vi "Subvi sample and hold bool.vi"(6 "Reset":bool, 8 "Refresh":bool, 9 "Input":bool) -> (1 "Output":bool)   [LabVIEW 2017]
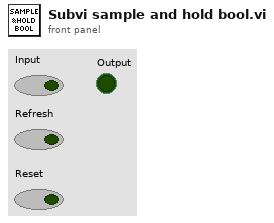
[diagram p1: front panel]
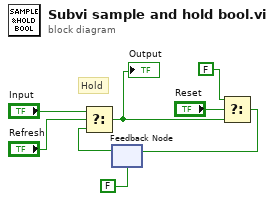
[diagram p0: block diagram]
diagram:
  # "Hold"
  n1 = feedback #1(FALSE) -> (w7:bool)
  n2 = Select(t="Input", s="Refresh", f=w7) -> (s? t:f=w3:bool)
  "Output" <- w3
  n3 = Select(t=FALSE, s="Reset", f=w3) -> (s? t:f=w6:bool)
  n4 = feedback-in #1(w6) -> ()
